vi "Set Log Config.vi"(8 "error in (no error)":errorcluster, 11 "Log Config":T1={"Log Level"=enum."WARNING"}) -> (0 "error out":errorcluster)   [LabVIEW 2020, in "RxnRover.lvlib" / "logging.lvlib"]
doc: "Sets the logging configuration."
uses:
  logging.lvlib
  Log Config.ctl
  Log Levels.ctl
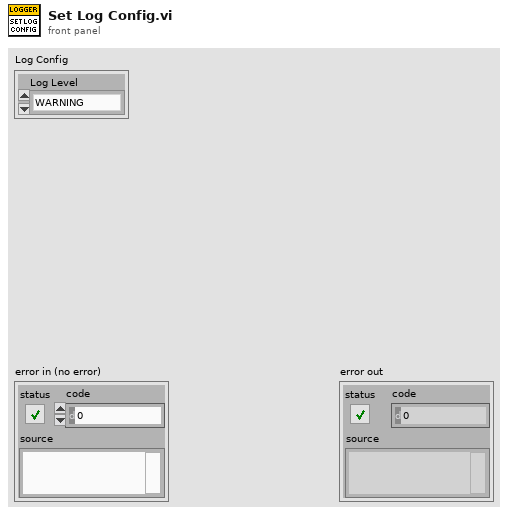
[diagram p1: front panel]
types:
  T1 = typedef "RxnRover.lvlib/logging.lvlib/Log Config.ctl" = cluster{"Log Level":T2}
  T2 = typedef "RxnRover.lvlib/logging.lvlib/Log Levels.ctl" = enum16{"NOTSET", "DEBUG", "INFO", "WARNING", "ERROR", "CRITICAL"}
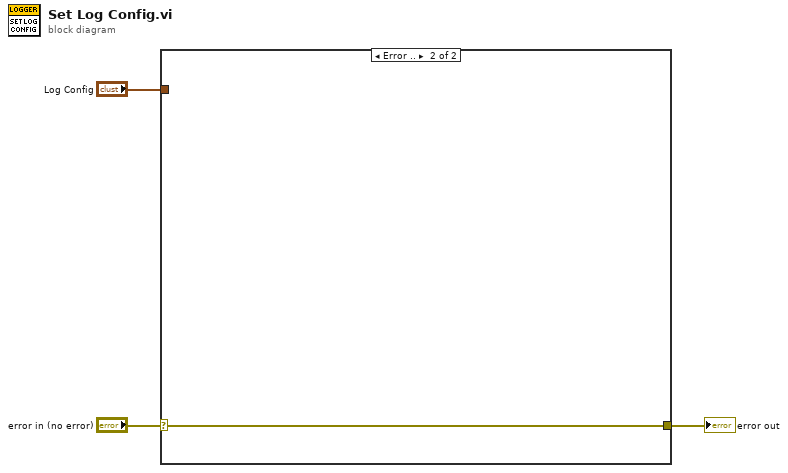
[diagram p0: block diagram]
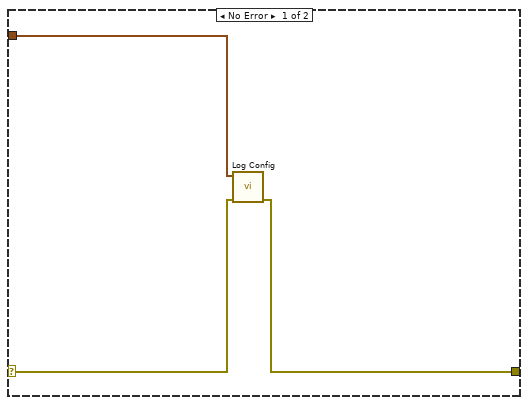
[diagram p2: hidden frame]
diagram:
  n1 = case shown="Error .." "error in (no error)" {
    selector: "error in (no error)" -> [w6 w7]
    tunnel: [w5 w7] -> w2
    tunnel: "Log Config" -> [w4 _]
    frame No Error {
      n2 = call "Log Config.vi"("error in (no error)"=w6, "Log Config in"=w4) -> ("error out"=w5:errorcluster)  [unwired: 8 in, 1 out]
    }
    frame Error {
    }
  }
  "error out" <- w2
